vi "Pcre2PatternInfoNameCount8.vi"(8 "error in":errorcluster, 11 "pCode":u64 format="%.0x") -> (0 "error out":errorcluster, 2 "NameCount":i32, 3 "pCode":u64 format="%.0x")   [LabVIEW 2021, in "libpcre2-8.lvlib"]
uses:
  libpcre2-8.lvlib
  Pcre2FnkCallError.vi
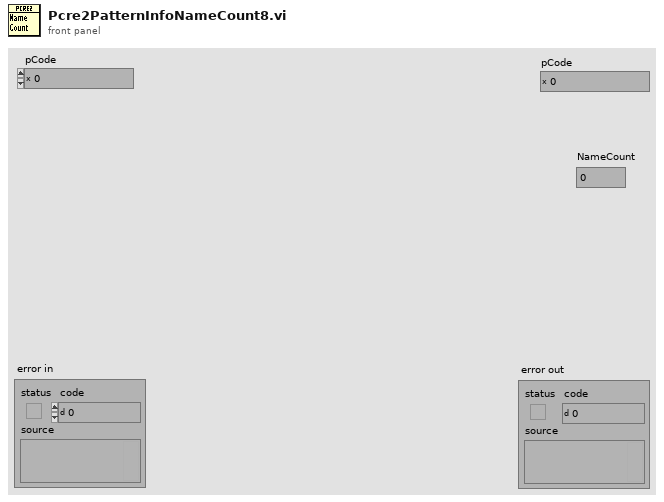
[diagram p1: front panel]
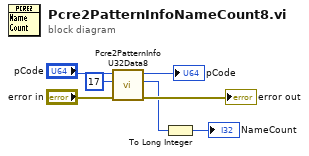
[diagram p0: block diagram]
diagram:
  n1 = call "Pcre2PatternInfoU32Data8.vi"("error in"="error in", "What"=u32 17, "pCode"="pCode") -> ("error out"=→"error out":errorcluster, "Info"=w2:u32, "pCode"=→"pCode":u64)  [unwired: 6 in]
  n2 = To Long Integer(number=w2) -> (32bit integer=→"NameCount":i32)
